vi "FSK_Deconvcode.vi"(8 "error in (no error)":errorcluster caption="错误输入（无错误）", 10 "RecvDeSync":dbl[](array[numeric]), 11 "PathIn":path) -> (0 "error out":errorcluster caption="错误输出", 2 "RecvBit":dbl[](array[numeric]) format="%#_13g", 3 "PathOut":path)   [LabVIEW 2015]
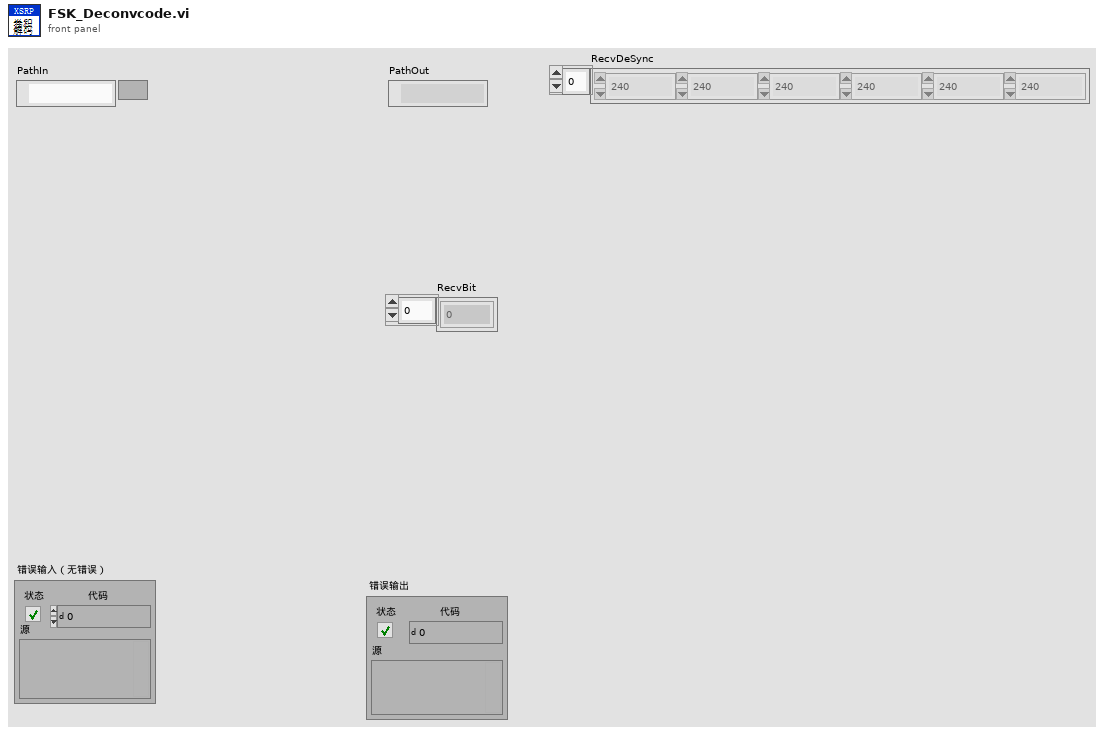
[diagram p1: front panel]
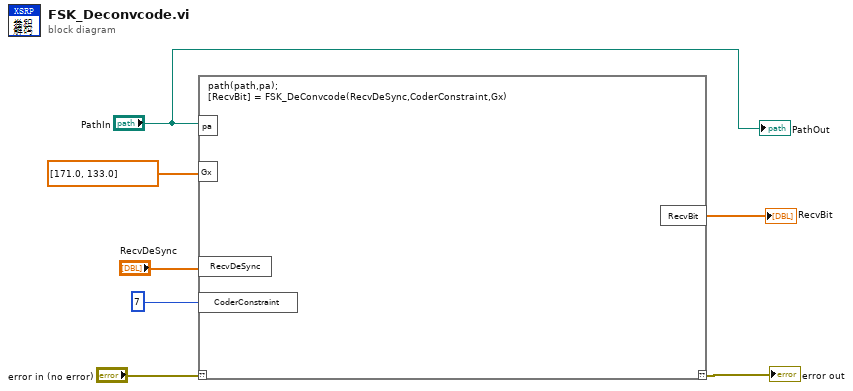
[diagram p0: block diagram]
diagram:
  n1 = script code="path(path,pa);\n[RecvBit] = FSK_DeConvcode(RecvDeSync,CoderConstraint,Gx)"("??"="error in (no error)", "pa"="PathIn", "RecvDeSync"="RecvDeSync", "CoderConstraint"=7, "Gx"=dbl[] [171.0, 133.0]) -> ("??"=→"error out":errorcluster, "RecvBit"=→"RecvBit":dbl[])
  "PathOut" <- "PathIn"
